vi "FlatToRichgrpc_reflection_v1alpha_ExtensionNumberResponse.vi"(5 "OutputClusterType":T1, 11 "InputCluster":T2) -> (3 "OutputCluster":T1)   [LabVIEW 2025, in "reflection_server.lvlib"]
uses:
  reflection_server.lvlib
  grpc_reflection_v1alpha_ExtensionNumberResponse_Flat.ctl
  grpc_reflection_v1alpha_ExtensionNumberResponse.ctl
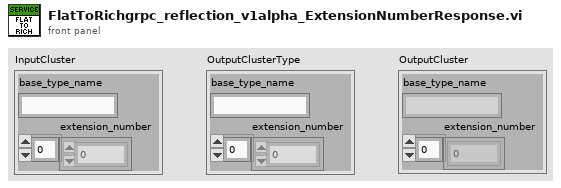
[diagram p1: front panel]
types:
  T1 = typedef "reflection_server.lvlib/grpc_reflection_v1alpha_ExtensionNumberResponse.ctl" = cluster{"base_type_name":string, "extension_number":i32[]}
  T2 = typedef "reflection_server.lvlib/grpc_reflection_v1alpha_ExtensionNumberResponse_Flat.ctl" = cluster{"base_type_name":string, "extension_number":i32[]}
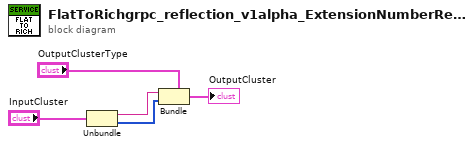
[diagram p0: block diagram]
diagram:
  n1 = Unbundle "Unbundle"("InputCluster") -> ("base_type_name"=w2:string, "extension_number"=w1:i32[])
  n2 = Bundle "Bundle"(cluster="OutputClusterType", "base_type_name"=w2, "extension_number"=w1) -> (→"OutputCluster":T1)
